vi "Addition of CP (SubVI).vi"(1 "ifft_output":cdb[](array[numeric]), 2 "cp_length":i16) -> (0 "ifft_output with CP":cdb[](array[numeric]))   [LabVIEW 2015]
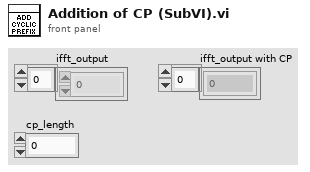
[diagram p1: front panel]
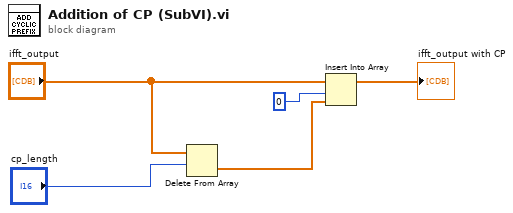
[diagram p0: block diagram]
diagram:
  n1 = Delete From Array(array="ifft_output", length="cp_length") -> (deleted portion=w4:cdb[])  [unwired: 1 in, 1 out]
  n2 = Insert Into Array(array="ifft_output", index=0, new element=w4) -> (→"ifft_output with CP":cdb[])
